vi "Stop Core.vi"(10 "final error code":i32, 11 "Command in":refnum<class "Command Actor.lvclass">) -> (3 "Command out":refnum<class "Command Actor.lvclass">)   [LabVIEW 2014, in "Robot Actor Framework.lvlib" / "Command Actor.lvlib" / "Command Actor.lvclass"]
doc: "(<B>Filename</B>: Actor Framework.lvlib:Actor.lvclass:Stop Core.vi)\n\nDefines what the actor does before it stops. Use the <B>final error code</B> input to determine whether the actor shut down in response to an error.\n\nBy default, this method does nothing. A descendant class may override it to define behavior, such as shutting down any processes the actor initiated in its override of the Actor Core method."
uses:
  Command Actor.lvclass
  <vilib>/ActorFramework/Message Enqueuer/Message Priority.ctl
  <vilib>/ActorFramework/Actor/Actor.lvclass/Actor.ctl
  Command Actor.lvclass/Command Actor.ctl
  Command Processor Actor/Command Processor Actor Messages/Command Stopped Msg/Command Stopped Msg.lvclass/Command Stopped Msg.ctl
  <vilib>/ActorFramework/Message Enqueuer/Message Enqueuer.lvclass/Message Enqueuer.ctl
  <vilib>/ActorFramework/Message Enqueuer/Enqueue.vi
  <vilib>/ActorFramework/Message Priority Queue/Priority Enqueue.vi
  Command Processor Actor/Command Processor Actor Messages/Command Stopped Msg/Command Stopped Msg.lvclass
  <vilib>/ni/Actors/State Actor/State Actor/State Actor.lvclass
  <vilib>/ActorFramework/Actor/Actor.lvclass
  <vilib>/ActorFramework/Message Enqueuer/Message Enqueuer.lvclass
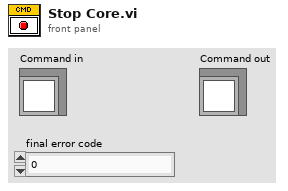
[diagram p1: front panel]
types:
  T1 = typedef "Actor Framework.lvlib/Message Enqueuer.lvclass/Message Priority.ctl" = enum16{"Low", "Normal", "High"}
  T2 = enum16{"Critical", "Error", "Warning", "Informational", "Debug"}
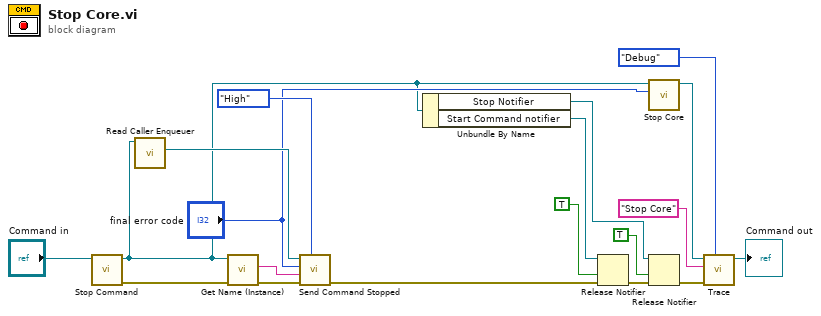
[diagram p0: block diagram]
diagram:
  n1 = call-dynamic "Stop Command.vi"("Command Actor in"="Command in") -> ("error out"=w3:errorcluster, "Command Actor out"=w6:refnum<class "Command Actor.lvclass">)  [unwired: 9 in]
  n2 = call <vilib>:"Read Caller Enqueuer.vi"("Actor"=w6) -> ("Caller Enqueuer"=w18:refnum<class "Message Enqueuer.lvclass">)  [unwired: 10 in]
  n3 = call-dynamic "Get Name (Instance).vi"("error in (no error)"=w3, "Command Actor in"=w6) -> ("error out"=w2:errorcluster, "Name (Instance)"=w15:string)  [unwired: 7 in, 1 out]
  n4 = call "Send Command Stopped.vi"("Message Priority (Normal)"=Message_Priority."High", "error in (no error)"=w2, "Command Name (Instance)"=w15, "final error code"="final error code", "Message Enqueuer"=w18) -> ("error out"=w1:errorcluster)  [unwired: 5 in, 1 out]
  n5 = Unbundle By Name(w6) -> ("Stop Notifier"=w19:refnum<notifier>, "Start Command notifier"=w13:refnum<notifier>)
  n6 = Release Notifier(notifier=w13, force destroy? (F)=TRUE, error in (no error)=w1) -> (error out=w5:errorcluster)  [unwired: 2 out]
  n7 = call-parent "Stop Core.vi"("final error code"="final error code", "Actor in"=w6) -> ("Actor out"=w8:refnum<class "Command Actor.lvclass">)  [unwired: 9 in]
  n8 = Release Notifier(notifier=w19, force destroy? (F)=TRUE, error in (no error)=w5) -> (error out=w4:errorcluster)  [unwired: 2 out]
  n9 = call-dynamic "Trace.vi"("Trace Level"=T2."Debug", "error in (no error)"=w4, "Command Action"="Stop Core" ("Trace Message"), "Command Actor in"=w8) -> ("Command Actor out"=→"Command out":refnum<class "Command Actor.lvclass">)  [unwired: 6 in, 1 out]
